vi "WriteStart.vi"(8 "error in (no error)":errorcluster, 9 "Cmd":u8, 10 "Address":u8, 11 "VISA Refnum in":refnum<visa-resource-name>) -> (0 "error out":errorcluster, 2 "String Out":string, 3 "VISA Refnum out":refnum<visa-resource-name>)   [LabVIEW 2015, in "Ion Motion Roboclaw.lvlib"]
uses:
  <instrlib>/Ion Motion Roboclaw/Ion Motion Roboclaw.lvlib
  <vilib>/Instr/_visa.llb/VISA Flush IO Buffer Mask.ctl
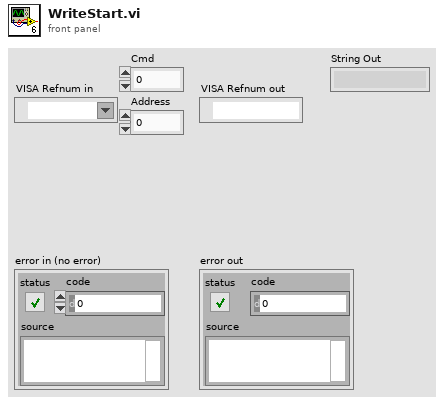
[diagram p1: front panel]
types:
  T1 = typedef "VISA Flush IO Buffer Mask.ctl" = u16
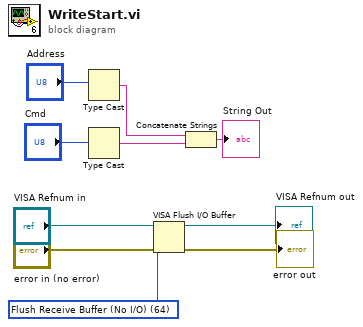
[diagram p0: block diagram]
diagram:
  w8 = T1 64 items=["Flush Receive Buffer"=16, "Write Transmit Buffer to Device"=32, "Flush Receive Buffer (No I/O)"=64, "Flush Transmit Buffer"=128] ("Mask")
  n1 = Type Cast(x="Address") -> (*(type *) &x=w1:string)  [unwired: 1 in]
  n2 = Type Cast(x="Cmd") -> (*(type *) &x=w3:string)  [unwired: 1 in]
  n3 = VISA Flush I/O Buffer(VISA resource name="VISA Refnum in", mask (16)=w8, error in (no error)="error in (no error)") -> (VISA resource name out=→"VISA Refnum out":refnum<visa-resource-name>, error out=→"error out":errorcluster)
  n4 = Concatenate Strings(w1, w3) -> (→"String Out":string)
